vi "Display n or dt.vi"(9 "Display n?":bool, 11 "Input Waveforms":waveform(dbl)[](array[waveform])) -> (3 "Output Waveforms":waveform(dbl)[](array[waveform]))   [LabVIEW 2016]
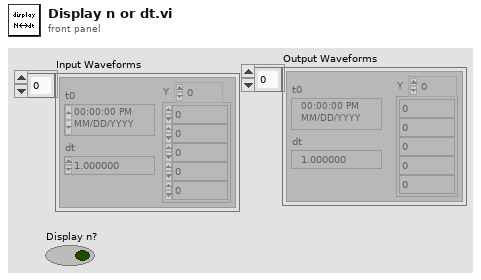
[diagram p1: front panel]
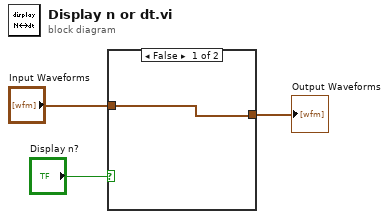
[diagram p0: block diagram]
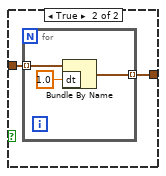
[diagram p2: hidden frame]
diagram:
  n1 = case shown="False" "Display n?" {
    tunnel: [w4 w6] -> w3
    tunnel: "Input Waveforms" -> [w4 w5]
    frame False {
    }
    frame True {
      n2 = for {
        tunnel: [w9] -> w6 mode=indexing
        tunnel: w5 -> [w8] mode=indexing
        n3 = Bundle By Name(cluster=w8, "dt"=1.0) -> (w9:waveform(dbl))
      }
    }
  }
  "Output Waveforms" <- w3
